vi "Simple Edge Counting - Gated.vi"() -> ()   [LabVIEW 2009]
uses:
  <vilib>/DAQmx/create/channels.llb/DAQmx Create Channel (CI-Count Edges).vi
  <vilib>/DAQmx/read.llb/DAQmx Read (Counter DBL 1Chan 1Samp).vi
  Program Files/National Instruments/LabVIEW 2009/resource/objmgr/daqmx.rc
panel:
  in  "Pause.DigLvl.When":i32(ring)=10214 items=["High"=10192, "Low"=10214]
  in  "Pause.DigLvl.Src":tag
  in  "Pause.TrigType":i32(ring)=10152 items=["Analog Level"=10101, "Analog Window"=10103, "Digital Level"=10152, "None"=10230]
  in  "stop":bool
  out "Count":dbl format="%0.2f"
  in  "count direction":i32(ring)=10128 items=["Count Up"=10128, "Count Down"=10124, "Externally Controlled"=10326]
  in  "initial count":u32
  in  "counter":tag
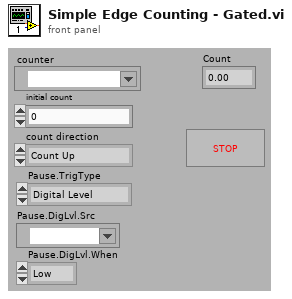
[diagram p1: front panel]
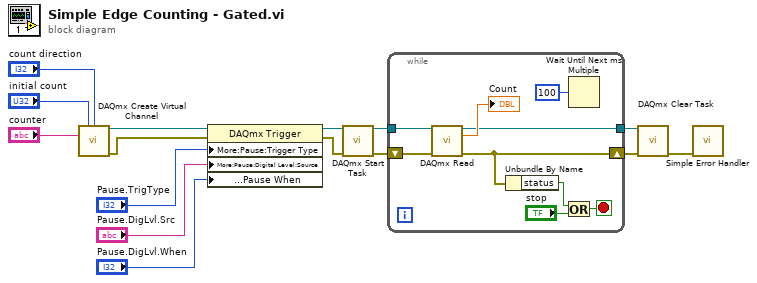
[diagram p0: block diagram]
diagram:
  n1 = call-poly <vilib>:"DAQmx Create Virtual Channel.vi"("initial count"="initial count", "count direction"="count direction", "counter"="counter") -> ("task out"=w7:refnum<k21>, "error out"=w4:errorcluster)  [unwired: 11 in]
  n2 = property on="Property Node" class="DAQmx Trigger"(reference=w7, error in=w4, "More:Pause:Trigger Type"="Pause.TrigType", "More:Pause:Digital Level:Source"="Pause.DigLvl.Src", "More:Pause:Digital Level:Pause When"="Pause.DigLvl.When") -> (reference out=w6:refnum<k21>, error out=w5:errorcluster)
  n3 = call <vilib>:"DAQmx Start Task.vi"("task/channels in"=w6, "error in"=w5) -> ("task out"=w12:refnum<k21>, "error out"=w11:errorcluster)  [unwired: 12 in]
  n4 = while {
    tunnel: w12 -> [w24]
    tunnel: [w21] -> w10
    shift-right: [w20] -> w9
    shift-left: w11 -> [w23]
    stop <- w17 stop-if-true
    n5 = call-poly <vilib>:"DAQmx Read.vi"("task/channels in"=w24, "error in"=w23) -> ("task out"=w21:refnum<k21>, "data"=→"Count":dbl, "error out"=w20:errorcluster)  [unwired: 11 in]
    n6 = Unbundle By Name "Unbundle By Name"(w20) -> ("status"=w19:bool)
    n7 = Or(x=w19, y="stop") -> (x .or. y?=w17:bool)
    n8 = Wait Until Next ms Multiple(millisecond multiple=u32 100) -> ()  [unwired: 1 out]
  }
  n9 = call <vilib>:"DAQmx Clear Task.vi"("task in"=w10, "error in"=w9) -> ("error out"=w8:errorcluster)  [unwired: 13 in]
  n10 = call <vilib>:"Simple Error Handler.vi"("error in (no error)"=w8) -> ()  [unwired: 4 in, 5 out]
